vi "Configure Ramp Down Time.vi"(0 "VISA resource name":refnum<visa-resource-name>, 5 "Ramp Down Time (0 s)":dbl min=0.0 max=999.9 format="%.1f", 11 "error in (no error)":errorcluster) -> (4 "VISA resource name out":refnum<visa-resource-name>, 15 "error out":errorcluster)   [LabVIEW 2014, in "eec 6700.lvlib"]
doc: "Sets the <B>Ramp down time</B> in the power source instrument.\n\n<B>Range</B> : 0~999.9 s\n\nThe ramp down parameter configures a time duration in which the output voltage is reduced to zero after the dwell time has completed."
uses:
  <instrlib>/eec 6700/eec 6700.lvlib
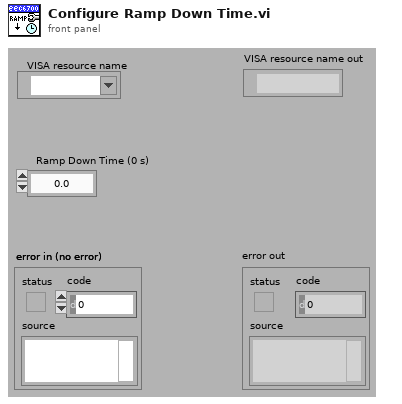
[diagram p1: front panel]
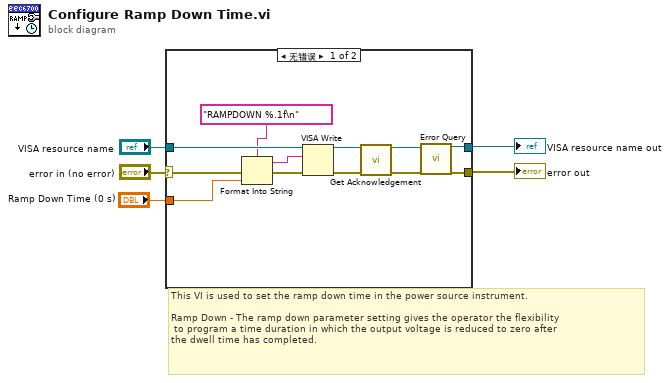
[diagram p0: block diagram]
diagram:
  # "This VI is used to set the ramp down time in the power source instrument. \n\nRamp Down - The ramp down parameter setting gives the operator the flexibility\n to program a time duration in which the output voltage is reduced to zero after \nthe dwell time has completed."
  n1 = case shown="无错误" "error in (no error)" {
    selector: "error in (no error)" -> [w11 w19]
    tunnel: "VISA resource name" -> [w17 w18]
    tunnel: [w13 w18] -> w4
    tunnel: [w12 w19] -> w3
    tunnel: "Ramp Down Time (0 s)" -> [w16 _]
    frame No Error {
      n2 = Format Into String(format string="RAMPDOWN %.1f\n" ("Command"), error in=w11, w16) -> (resulting string=w15:string, error out=w10:errorcluster)  [unwired: 1 in]
      n3 = VISA Write(VISA resource name=w17, write buffer=w15, error in (no error)=w10) -> (VISA resource name out=w7:refnum<visa-resource-name>, error out=w6:errorcluster)  [unwired: 1 out]
      n4 = call <instrlib>:"Get Acknowledgement.vi"("VISA resource name"=w7, "error in (no error)"=w6) -> ("VISA resource name out"=w8:refnum<visa-resource-name>, "error out"=w9:errorcluster)  [unwired: 12 in]
      n5 = call <instrlib>:"Error Query.vi"("VISA resource name"=w8, "error in (no error)"=w9) -> ("VISA resource name out"=w13:refnum<visa-resource-name>, "error out"=w12:errorcluster)  [unwired: 10 in, 2 out]
    }
    frame Error {
    }
  }
  "error out" <- w3
  "VISA resource name out" <- w4
